vi "Modules.vi"(7 "VI in":refnum<vi>, 8 "error in (no error)":errorcluster, 11 "Stop Event":refnum<user-event>) -> (0 "error out":errorcluster, 3 "User Event out":refnum<user-event>)   [LabVIEW 2020]
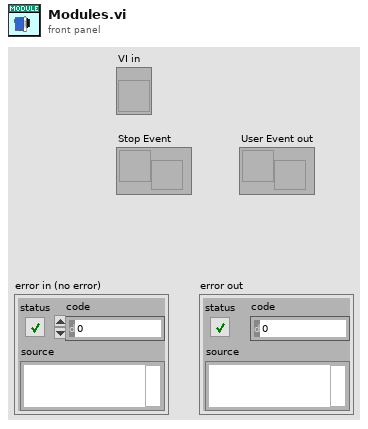
[diagram p1: front panel]
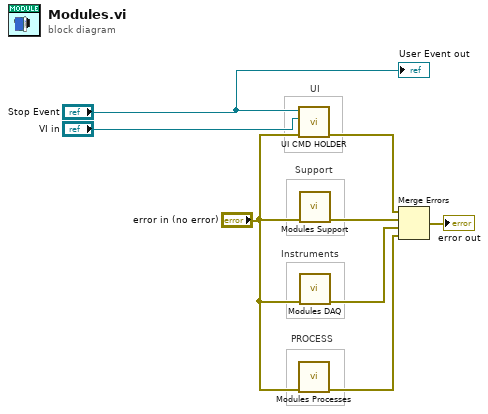
[diagram p0: block diagram]
diagram:
  # "UI"
  # "Instruments"
  # "Support"
  # "PROCESS"
  n1 = call "UI CMD HOLDER.vi"("error in (no error)"="error in (no error)", "VI in"="VI in", "Stop Event"="Stop Event") -> ("error out"=w5:errorcluster)  [unwired: 8 in]
  n2 = call "Modules Processes.vi"("error in (no error)"="error in (no error)") -> ("error out"=w1:errorcluster)  [unwired: 10 in]
  n3 = call "Modules Support.vi"("error in (no error)"="error in (no error)") -> ("error out"=w6:errorcluster)  [unwired: 10 in]
  n4 = call "Modules DAQ.vi"("error in (no error)"="error in (no error)") -> ("error out"=w7:errorcluster)  [unwired: 10 in]
  n5 = Merge Errors(w5, w6, w7, w1) -> (→"error out":errorcluster)
  "User Event out" <- "Stop Event"
